vi "DigitalOutCommand.vi"(2 "error in":errorcluster, 3 "Component ID":u16(ring) items=["left_itb_light_inner", "right_itb_light_inner", "torso_left_itb_light_inner", "torso_right_itb_light_inner", "left_itb_light_outer", "right_itb_light_outer", "torso_left_itb_light_outer", "torso_right_itb_light_outer", ""], 4 "State":bool, 5 "node":string) -> (0 "error out":errorcluster)   [LabVIEW 2010]
uses:
  ROS/Code/SubVIs/_ROSDirection.ctl
  ROS/Code/Console/Servers/ServerSubs/TopicDef.ctl
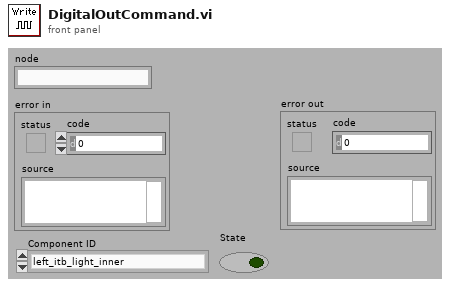
[diagram p1: front panel]
types:
  T1 = typedef "TopicDef.ctl" = cluster{"Topic":string, "Type":string, "Action":T2, "Update (ms)":u16, "write queue":u16}
  T2 = typedef "_ROSDirection.ctl" = enum16{"Node", "Publisher", "Subscriber", "Service Client"}
  T3 = typedef "_ROSControl.ctl" = cluster{"topic port":u16, "Node":string, "topic":string, "type":string, "node port":u32, "error ":errorcluster, "Direction":T2, "APIs":string[], "Update (ms)":u16, "write queue":u16}
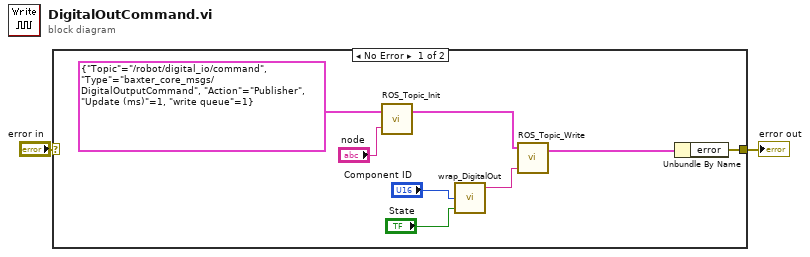
[diagram p0: block diagram]
diagram:
  n1 = case shown="No Error" "error in" {
    selector: "error in" -> [_ w11]
    tunnel: [w8 w11] -> w2
    frame No Error {
      n2 = call "ROS_Topic_Init.vi"("node"="node", "Definitions"=T1 {"Topic"="/robot/digital_io/command", "Type"="baxter_core_msgs/DigitalOutputCommand", "Action"=enum."Publisher", "Update (ms)"=1, "write queue"=1}) -> ("ROS out"=w10:T3)  [unwired: 1 in]
      n3 = call "wrap_DigitalOut.vi"("State"="State", "Component ID"="Component ID") -> ("msg out"=w6:string)  [unwired: 3 in]
      n4 = call "ROS_Topic_Write.vi"("Msg in"=w6, "ROS in"=w10) -> ("ROS out"=w9:T3)  [unwired: 2 in]
      n5 = Unbundle By Name(w9) -> ("error"=w8:errorcluster)
    }
    frame Error {
    }
  }
  "error out" <- w2
